vi "Test Subscriber.vi"() -> ()   [LabVIEW 2021]
uses:
  ChannelCommon/typedef/FIFO Config.ctl
  ChannelCommon/ChannelCommon.lvlib
  CIFChannels/Typedef/Direction.ctl
  CIFChannels/CIFChannels.lvclass
  CIF_NIChn_DAQ_Base.lvclass
  ChannelCommon/typedef/New FIFO Instance Response.ctl
  ChannelCommon/typedef/Datatype Waveform.ctl
panel:
  in  "stop":bool
  out "timed out?":bool
  out "DAQ Out":T1[](array[typedef])
  out "error out":errorcluster
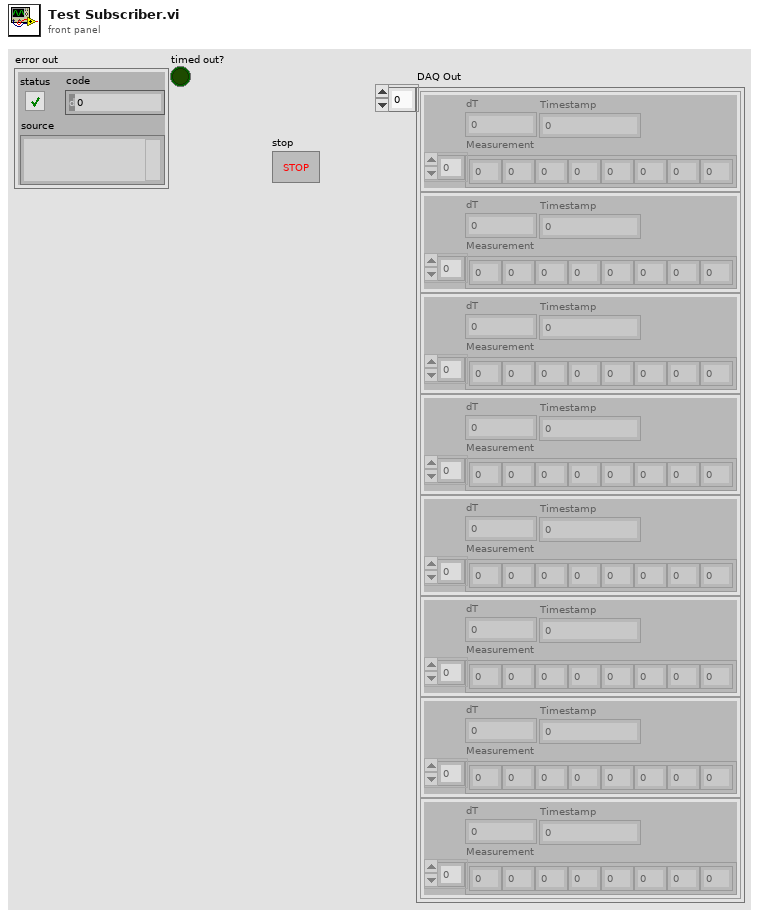
[diagram p1: front panel]
types:
  T1 = typedef "ChannelCommon.lvlib/Datatype Waveform.ctl" = cluster{"Measurement":dbl[], "dT":dbl, "Timestamp":i64}
  T2 = typedef "ChannelCommon.lvlib/New FIFO Instance Response.ctl" = cluster{"Publisher":string, "Custom Data":u8[]}
  T3 = typedef "ChannelCommon.lvlib/FIFO Config.ctl" = cluster{"Max Bytes/Msg":u64, "Max Msg/FIFO":u64, "Flags":u64}
  T4 = typedef "CIFChannels.lvclass/Direction.ctl" = enum16{"Publisher", "Subscriber"}
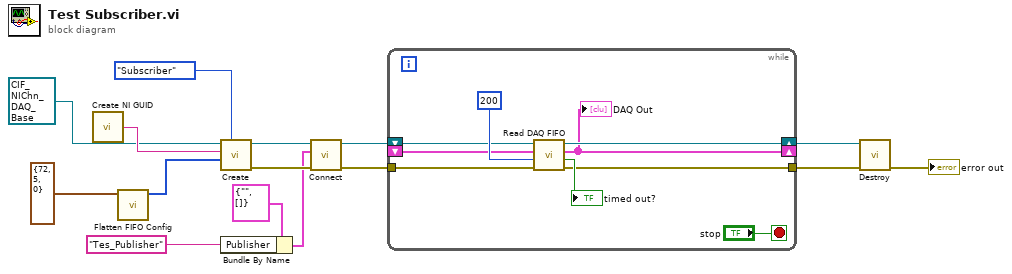
[diagram p0: block diagram]
diagram:
  n1 = call <vilib>:"Create NI GUID.vi"() -> ("NI GUID"=w10:string)
  n2 = call "Flatten FIFO Config.vi"("FIFO Config in"=T3 {"Max Bytes/Msg"=72, "Max Msg/FIFO"=5, "Flags"=0}) -> ("Flattened FIFO Config"=w5:u8[])  [unwired: 10 in]
  n3 = call-dynamic "Create.vi"("Direction"=Direction."Subscriber", "Custom Config Data"=w5, "Name"=w10, "CIF_NIChn_FIFO_DAQ in"=refnum<class "CIF_NIChn_DAQ_Base.lvclass"> refnum ("CIF_NIChn_FIFO_DAQ.lvclass")) -> ("error out"=w12:errorcluster, "CIF_NIChn_FIFO_DAQ out"=w13:refnum<class "CIF_NIChn_DAQ_Base.lvclass">)  [unwired: 6 in]
  n4 = Bundle By Name(cluster=T2 {"Publisher"="", "Custom Data"=[]} ("Connection"), "Publisher"="Tes_Publisher" ("Connection Name")) -> (w1:T2)
  n5 = call-dynamic "Connect.vi"("error in (no error)"=w12, "Connection"=w1, "CIFTag in"=w13) -> ("error out"=w7:errorcluster, "CIFTag out"=w9:refnum<class "CIF_NIChn_DAQ_Base.lvclass">)  [unwired: 7 in]
  n6 = while {
    shift-right: [w24] -> w15
    shift-left: w9 -> [w22]
    tunnel: w7 -> [w21]
    tunnel: [w19] -> w6
    shift-right: [w17] -> _
    shift-left: _ -> [w16]
    stop <- "stop" stop-if-true
    n7 = call-dynamic "Read DAQ FIFO.vi"("error in (no error)"=w21, "Timeout (ms)"=200, "Data In"=w16, "CIF_NIChn_FIFO_DAQ in"=w22) -> ("error out"=w19:errorcluster, "timed out?"=→"timed out?":bool, "Data Out"=w17:T1[], "CIF_NIChn_FIFO_DAQ out"=w24:refnum<class "CIF_NIChn_DAQ_Base.lvclass">)  [unwired: 3 in, 1 out]
    "DAQ Out" <- w17
  }
  n8 = call-dynamic "Destroy.vi"("error in (no error)"=w6, "CIF_NIChn_FIFO_DAQ in"=w15) -> ("error out"=→"error out":errorcluster)  [unwired: 8 in, 1 out]
